vi "Perform Action.vi"(7 "IPerform Action":refnum<class "Instrument.lvclass">, 8 "error in":errorcluster, 10 "Input":variant, 11 "Perform Action Red-y Read Write Strategy":refnum<class "Perform Action Red-y Read Write Strategy.lvclass">) -> (0 "error out":errorcluster, 2 "Output":variant, 3 "Virt Instrument Base out":refnum<class "Perform Action Red-y Read Write Strategy.lvclass">)   [LabVIEW 2023, in "Perform Action Red-y Read Write Strategy.lvclass"]
uses:
  Perform Action Red-y Read Write Strategy.lvclass
  Instrument/Instrument.lvclass
  Configurations/Pressure Control CFG/Read Write PE Input.ctl
  <userlib>/_OpenG.lib/lvdata/lvdata.llb/Type Descriptor Enumeration__ogtk.ctl
  Perform Action Red-y Read Write Strategy.lvclass/Perform Action Red-y Read Write Strategy.ctl
  <userlib>/_OpenG.lib/lvdata/lvdata.llb/openg_variant.lvlib
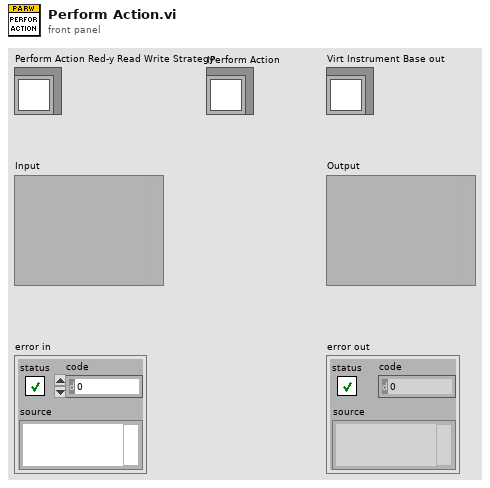
[diagram p1: front panel]
types:
  T1 = typedef "openg_variant.lvlib/Type Descriptor Enumeration__ogtk.ctl" = enum8{"<Null>", "I8", "I16", "I32", "I64", "U8", "U16", "U32", "U64", "SGL", "DBL", "EXT", "CSG", "CDB", "CXT", "0x0F", "0x10", "0x11", "0x12", "0x13", "0x14", "Enum U8", "Enum U16", "Enum U32", "Enum U64", "SGL PQ", "DBL PQ", "EXT PQ", "CSG PQ", "CDB PQ", "CXT PQ", "0x1F", "0x20", "Boolean", "0x22", "0x23", "0x24", "0x25", "0x26", "0x27", "0x28", "0x29", "0x2A", "0x2B", "0x2C", "0x2D", "0x2E", "0x2F", "String", "0x31", "Path", "Pict", "0x34", "0x35", "0x36", "DAQ", "0x38", "0x39", "0x3A", "0x3B", "0x3C", "0x3D", "0x3E", "0x3F", "Array", "0x41", "0x42", "0x43", "0x44", "0x45", "0x46", "0x47", "0x48", "0x49", "0x4A", "0x4B", "0x4C", "0x4D", "0x4E", "0x4F", "Cluster", "0x51", "0x52", "Variant", "Waveform", "0x55", "0x56", "0x57", "0x58", "0x59", "0x5A", "0x5B", "0x5C", "0x5D", "0x5E", "Fixed Point", "0x60", "0x61", "0x62", "0x63", "0x64", "0x65", "0x66", "0x67", "0x68", "0x69", "0x6A", "0x6B", "0x6C", "0x6D", "0x6E", "0x6F", "Refnum", "0x71", "0x72", "Set Collection", "Map Collection"}
  T2 = typedef "Read Write PE Input.ctl" = cluster{"Action":enum16{"Write", "Read"}, "Register":u16, "Type":T1, "Data":variant}
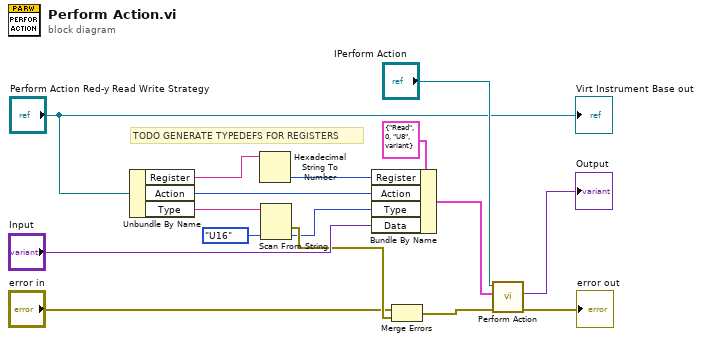
[diagram p0: block diagram]
diagram:
  # "TODO GENERATE TYPEDEFS FOR REGISTERS"
  n1 = Unbundle By Name("Perform Action Red-y Read Write Strategy") -> ("Register"=w5:string, "Action"=w6:enum16{"Write", "Read"}, "Type"=w11:string)
  n2 = Hexadecimal String To Number(string=w5) -> (number=w4:u32)  [unwired: 2 in, 1 out]
  n3 = Scan From String(input string=w11, default 1=Type_Descriptor_Enumeration__ogtk."U16" ("Type")) -> (error out=w8:errorcluster, output 1=w7:T1)  [unwired: 3 in, 2 out]
  n4 = Bundle By Name(cluster=T2 {"Action"=enum."Read", "Register"=0, "Type"=enum."U8", "Data"=variant} ("Cluster"), "Register"=w4, "Action"=w6, "Type"=w7, "Data"="Input") -> (w13:T2)
  n5 = Merge Errors("error in", w8) -> (w9:errorcluster)
  n6 = call "Perform Action.vi"("Error In"=w9, "Input"=w13, "reference in"="IPerform Action") -> ("Error Out"=→"error out":errorcluster, "Output"=→"Output":variant)  [unwired: 6 in, 1 out]
  "Virt Instrument Base out" <- "Perform Action Red-y Read Write Strategy"
